vi "GetProperties.vi"(8 "error in":errorcluster, 11 "Plot in":refnum<class "Plot.lvclass">) -> (0 "error out":errorcluster, 3 "Plot out":refnum<class "Plot.lvclass">)   [LabVIEW 2014, in "Raspberry Pi Compatible Compiler for LabVIEW.lvlib" / "Plot.lvclass"]
uses:
  Plot.lvclass
  Generic/Generic.lvclass/Generic.ctl
  Plot.lvclass/Plot.ctl
  Generic/Generic.lvclass
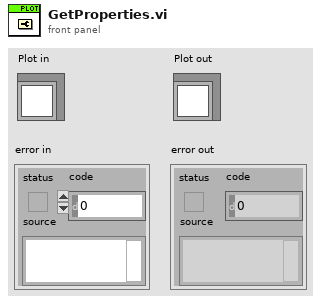
[diagram p1: front panel]
types:
  T1 = cluster{"Plot Color":u32, "Plot Interpolation":u8, "Point Style":u8, "Line Style":u8, "Fill/Pt. Color":u32, "Line Width":u8, "Bar Plot Style":u8, "Fill To":i16}
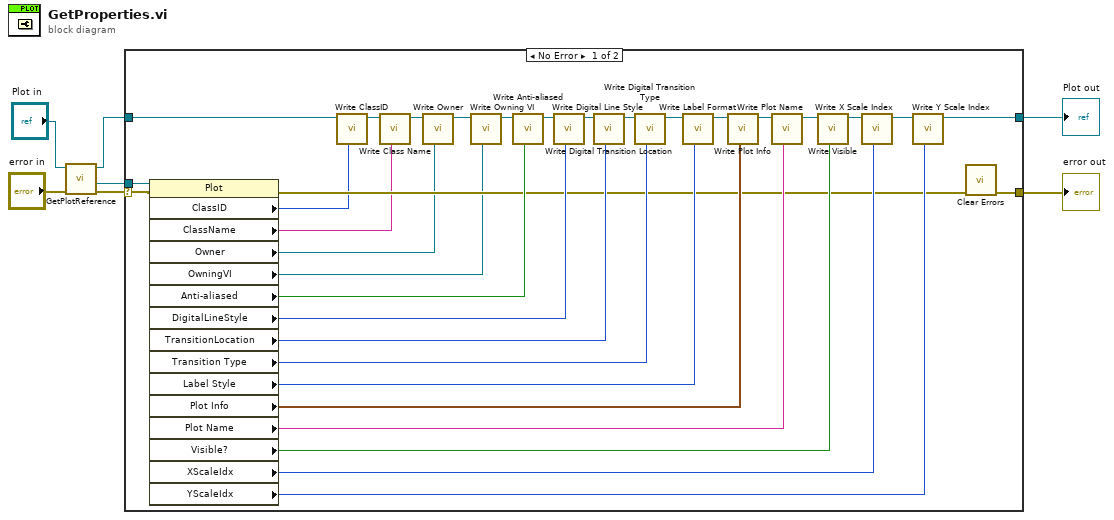
[diagram p0: block diagram]
diagram:
  n1 = call "GetPlotReference.vi"("error in"="error in", "Plot in"="Plot in") -> ("error out"=w7:errorcluster, "plot reference"=w6:refnum<vi>, "Plot out"=w5:refnum<class "Plot.lvclass">)  [unwired: 7 in]
  n2 = case shown="No Error" w7 {
    selector: w7 -> [w39 w42]
    tunnel: w6 -> [w40 _]
    tunnel: w5 -> [w13 w41]
    tunnel: [w20 w41] -> w4
    tunnel: [w17 w42] -> w3
    frame No Error {
      n3 = property class="Plot"(reference=w40, error in=w39) -> (error out=w18:errorcluster, "ClassID"=w11:u32, "ClassName"=w10:string, "Owner"=w9:refnum<vi>, "OwningVI"=w8:refnum<vi>, "Anti-aliased"=w38:bool, "DigitalLineStyle"=w36:u8, "TransitionLocation"=w35:u8, "Transition Type"=w32:u8, "Label Style"=w30:u8, "Plot Info"=w28:T1, "Plot Name"=w26:string, "Visible?"=w24:bool, "XScaleIdx"=w22:u32, "YScaleIdx"=w19:u32)  [unwired: 1 out]
      n4 = call "Write ClassID.vi"("ClassID"=w11, "Generic in"=w13) -> ("Generic out"=w14:refnum<class "Plot.lvclass">)  [unwired: 7 in]
      n5 = call "Write Class Name.vi"("Class Name"=w10, "Generic in"=w14) -> ("Generic out"=w15:refnum<class "Plot.lvclass">)  [unwired: 7 in]
      n6 = call "Write Owner.vi"("Owner"=w9, "Generic in"=w15) -> ("Generic out"=w16:refnum<class "Plot.lvclass">)  [unwired: 7 in]
      n7 = call "Write Owning VI.vi"("Owning VI"=w8, "Generic in"=w16) -> ("Generic out"=w12:refnum<class "Plot.lvclass">)  [unwired: 7 in]
      n8 = call "Write Anti-aliased.vi"("Anti-aliased"=w38, "Plot in"=w12) -> ("Plot out"=w37:refnum<class "Plot.lvclass">)  [unwired: 7 in]
      n9 = call "Write Digital Line Style.vi"("Digital Line Style"=w36, "Plot in"=w37) -> ("Plot out"=w34:refnum<class "Plot.lvclass">)  [unwired: 7 in]
      n10 = call "Write Digital Transition Location.vi"("Digital Transition Location"=w35, "Plot in"=w34) -> ("Plot out"=w33:refnum<class "Plot.lvclass">)  [unwired: 7 in]
      n11 = call "Write Digital Transition Type.vi"("Digital Transition Type"=w32, "Plot in"=w33) -> ("Plot out"=w31:refnum<class "Plot.lvclass">)  [unwired: 7 in]
      n12 = call "Write Label Format.vi"("Label Format"=w30, "Plot in"=w31) -> ("Plot out"=w29:refnum<class "Plot.lvclass">)  [unwired: 7 in]
      n13 = call "Write Plot Info.vi"("Plot Info"=w28, "Plot in"=w29) -> ("Plot out"=w27:refnum<class "Plot.lvclass">)  [unwired: 7 in]
      n14 = call "Write Plot Name.vi"("Plot Name"=w26, "Plot in"=w27) -> ("Plot out"=w25:refnum<class "Plot.lvclass">)  [unwired: 7 in]
      n15 = call "Write Visible.vi"("Visible"=w24, "Plot in"=w25) -> ("Plot out"=w23:refnum<class "Plot.lvclass">)  [unwired: 7 in]
      n16 = call "Write X Scale Index.vi"("X Scale Index"=w22, "Plot in"=w23) -> ("Plot out"=w21:refnum<class "Plot.lvclass">)  [unwired: 7 in]
      n17 = call "Write Y Scale Index.vi"("Y Scale Index"=w19, "Plot in"=w21) -> ("Plot out"=w20:refnum<class "Plot.lvclass">)  [unwired: 7 in]
      n18 = call <vilib>:"Clear Errors.vi"("error in (no error)"=w18) -> ("error out"=w17:errorcluster)  [unwired: 5 in, 1 out]
    }
    frame Error {
    }
  }
  "error out" <- w3
  "Plot out" <- w4
